vi "Global Name Set.vi"(8 "error in (no error)":errorcluster, 10 "Name":string, 11 "Name Actions":T1) -> (0 "error out":errorcluster, 1 "All Names":string[](array[string]), 2 "Index":i32)   [LabVIEW 2009]
uses:
  Name Actions.ctl
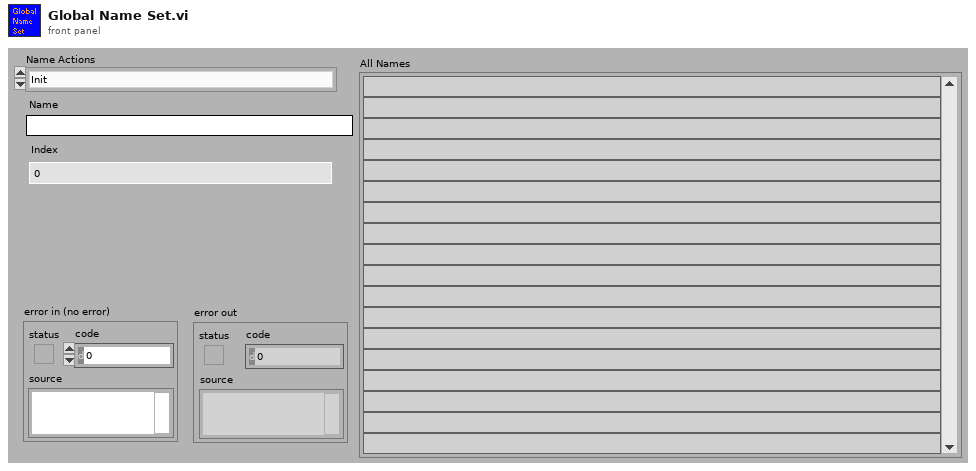
[diagram p1: front panel]
types:
  T1 = typedef "Name Actions.ctl" = enum16{"Init", "Get Names", "Get Index"}
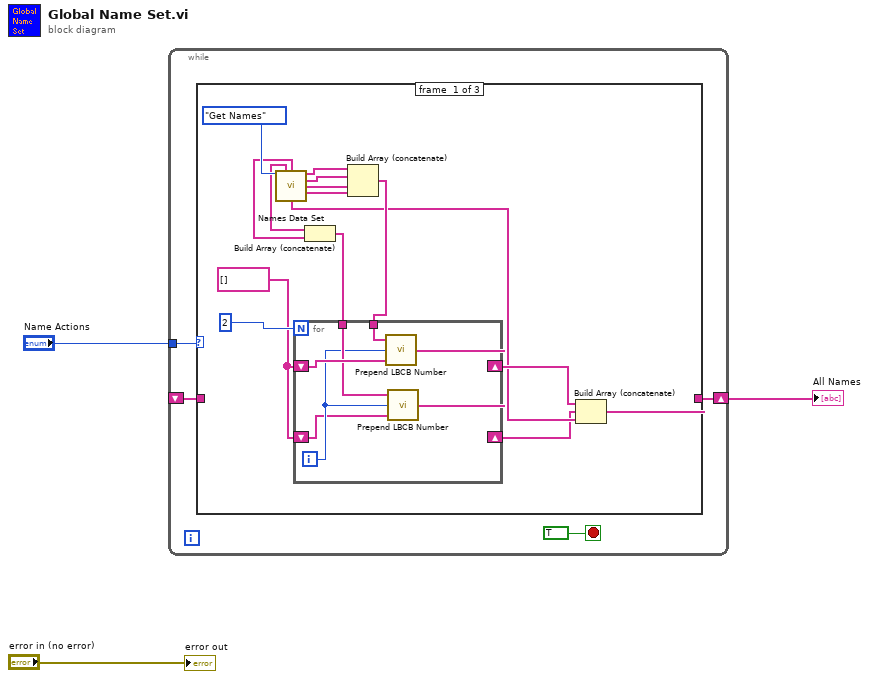
[diagram p0: block diagram]
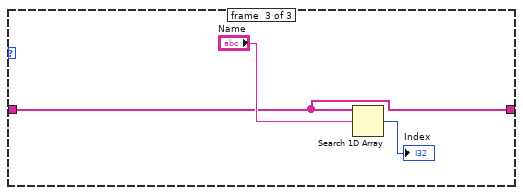
[diagram p3: hidden frame]
diagram:
  n1 = while {
    tunnel: "Name Actions" -> [w6]
    shift-right: [w5] -> w1
    shift-left: _ -> [w4]
    stop <- TRUE stop-if-true
    n2 = case shown="\"Get Index\"" w6 {
      tunnel: [w17 w30 w31] -> w5
      tunnel: w4 -> [_ w30 w31]
      frame #0 {
        w10 = string[] [] ("Prepended Out")
        n3 = call "Names Data Set.vi"("Name Actions"=Name_Actions."Get Names") -> ("Actuator Command Volts"=w13:string[], "Actuator Volt Readings"=w12:string[], "Cartesian Commands"=w22:string[], "Cartesian Readings"=w21:string[], "Actuator Commands"=w20:string[], "Actuator Readings"=w19:string[], "External Sensor Names"=w9:string[])  [unwired: 1 in, 7 out]
        n4 = Build Array (concatenate)(w13, w12) -> (w11:string[])
        n5 = Build Array (concatenate)(w22, w21, w20, w19) -> (w16:string[])
        n6 = for {
          N: 2 -> [_]
          shift-right: [w27] -> w15
          shift-left: w10 -> [w28]
          tunnel: w16 -> [w29]
          tunnel: w11 -> [w26]
          shift-right: [w24] -> w8
          shift-left: w10 -> [w23]
          i -> [w25]
          n7 = call "Prepend LBCB Number.vi"("Prepended In"=w28, "LBCB Number"=w25, "Names In"=w29) -> ("Prepended Out"=w27:string[])
          n8 = call "Prepend LBCB Number.vi"("Prepended In"=w23, "LBCB Number"=w25, "Names In"=w26) -> ("Prepended Out"=w24:string[])
        }
        n9 = Build Array (concatenate)(w15, w8, w9) -> (w17:string[])
      }
      frame #1 {
      }
      frame #2 {
        n10 = Search 1D Array(1D array=w31, element="Name") -> (index of element=→"Index":i32)  [unwired: 1 out]
      }
    }
  }
  "All Names" <- w1
  "error out" <- "error in (no error)"
